vi "SubVi.Reading data from an ini file.vi"(5 "Data in the cluster":T2, 7 "Source file":path) -> (0 "error out":errorcluster, 3 "Array":T1(array[cluster]))   [LabVIEW 2015]
doc: "Reads data from an ini file"
uses:
  <vilib>/Utility/config.llb/Read Key (String).vi
  <vilib>/Utility/config.llb/NI_LVConfig.lvlib
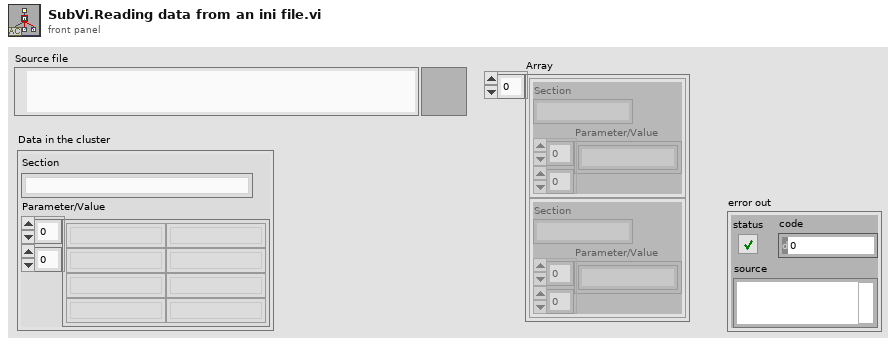
[diagram p1: front panel]
types:
  T1 = cluster{"Section":string, "Parameter/Value":string[][]}[]
  T2 = cluster{"Section":string, "Parameter/Value":string[][]}
  T3 = typedef "NI_LVConfig.lvlib/Config Data RefNum.ctl" = refnum<k1>
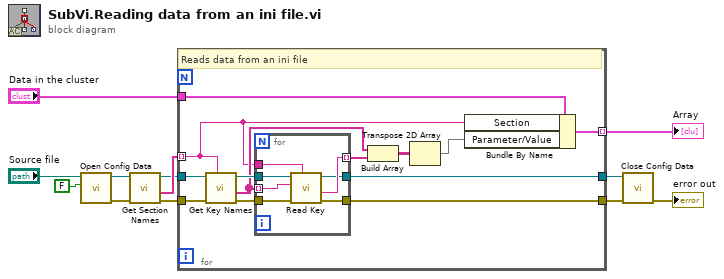
[diagram p0: block diagram]
diagram:
  n1 = call <vilib>:"Open Config Data.vi"("create file if necessary (T)"=FALSE, "configuration file path"="Source file") -> ("error out"=w2:errorcluster, "refnum"=w1:T3)  [unwired: 7 in, 1 out]
  n2 = call <vilib>:"Get Section Names.vi"("error in (no error)"=w2, "refnum"=w1) -> ("error out"=w4:errorcluster, "section names"=w5:string[], "refnum out"=w3:T3)  [unwired: 7 in]
  n3 = for {
    tunnel: w5 -> [w18] mode=indexing
    tunnel: w3 -> [w24]
    tunnel: w4 -> [w25]
    tunnel: [w17] -> w10 mode=indexing
    tunnel: "Data in the cluster" -> [w16]
    tunnel: [w14] -> w11
    tunnel: [w13] -> w8
    # "Reads data from an ini file"
    n4 = call <vilib>:"Get Key Names.vi"("section"=w18, "error in (no error)"=w25, "refnum"=w24) -> ("error out"=w23:errorcluster, "key names"=w21:string[], "refnum out"=w22:T3)  [unwired: 5 in, 1 out]
    n5 = for {
      tunnel: w18 -> [w32]
      tunnel: w21 -> [w31] mode=indexing
      tunnel: w22 -> [w30]
      tunnel: w23 -> [w29]
      tunnel: [w28] -> w20 mode=indexing
      tunnel: [w27] -> w13
      tunnel: [w26] -> w14
      n6 = call-poly <vilib>:"Read Key.vi"("section"=w32, "error in (no error)"=w29, "key"=w31, "refnum"=w30) -> ("error out"=w26:errorcluster, "value"=w28:string, "refnum out"=w27:T3)  [unwired: 4 in, 1 out]
    }
    n7 = Build Array(w21, w20) -> (w19:string[][])
    n8 = Transpose 2D Array(2D array=w19) -> (transposed array=w15:string[][])
    n9 = Bundle By Name(cluster=w16, "Section"=w18, "Parameter/Value"=w15) -> (w17:T2)
  }
  "Array" <- w10
  n10 = call <vilib>:"Close Config Data.vi"("error in (no error)"=w11, "refnum"=w8) -> ("error out"=→"error out":errorcluster)  [unwired: 8 in, 1 out]
